vi "Non_empty_judgment.vi"(0 "TEMP":string, 1 "HN":string[](array[string]), 2 "生产日期":string, 3 "校准日期":string, 4 "核验员":string, 5 "HS":sgl[](array[numeric]), 6 "MODE":string, 7 "TV":sgl[][](array[numeric]), 8 "DIN":string, 9 "TESTS":sgl[][](array[numeric]), 10 "TSN":string, 11 "NAME":string) -> (16 "结果":bool)   [LabVIEW 2019]
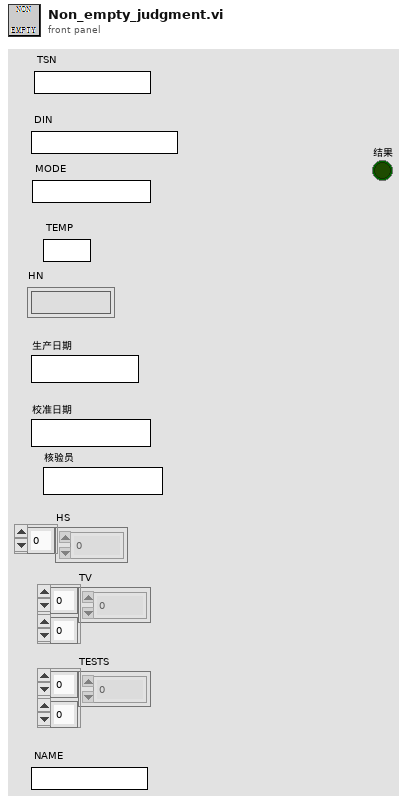
[diagram p1: front panel]
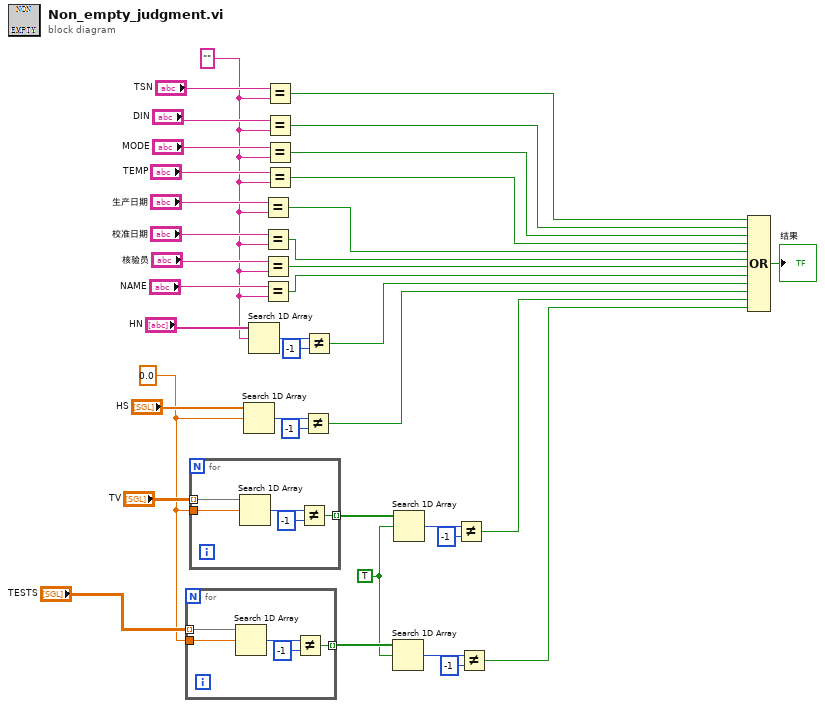
[diagram p0: block diagram]
diagram:
  w18 = TRUE
  w21 = 0.0
  w29 = ""
  n1 = for {
    tunnel: "TESTS" -> [w41] mode=indexing
    tunnel: w21 -> [w40]
    tunnel: [w39] -> w19 mode=indexing
    n2 = Search 1D Array(1D array=w41, element=w40) -> (index of element=w42:i32)  [unwired: 1 in]
    n3 = Not Equal?(x=w42, y=-1) -> (x != y?=w39:bool)
  }
  n4 = for {
    tunnel: "TV" -> [w46] mode=indexing
    tunnel: w21 -> [w45]
    tunnel: [w44] -> w20 mode=indexing
    n5 = Search 1D Array(1D array=w46, element=w45) -> (index of element=w47:i32)  [unwired: 1 in]
    n6 = Not Equal?(x=w47, y=-1) -> (x != y?=w44:bool)
  }
  n7 = Search 1D Array(1D array="HS", element=w21) -> (index of element=w24:i32)  [unwired: 1 in]
  n8 = Search 1D Array(1D array="HN", element=w29) -> (index of element=w28:i32)  [unwired: 1 in]
  n9 = Equal?(x="生产日期", y=w29) -> (x = y?=w9:bool)
  n10 = Equal?(x="校准日期", y=w29) -> (x = y?=w8:bool)
  n11 = Equal?(x="核验员", y=w29) -> (x = y?=w7:bool)
  n12 = Equal?(x="NAME", y=w29) -> (x = y?=w6:bool)
  n13 = Equal?(x="TSN", y=w29) -> (x = y?=w13:bool)
  n14 = Equal?(x="DIN", y=w29) -> (x = y?=w12:bool)
  n15 = Equal?(x="MODE", y=w29) -> (x = y?=w11:bool)
  n16 = Equal?(x="TEMP", y=w29) -> (x = y?=w10:bool)
  n17 = Not Equal?(x=w24, y=-1) -> (x != y?=w4:bool)
  n18 = Not Equal?(x=w28, y=-1) -> (x != y?=w5:bool)
  n19 = Search 1D Array(1D array=w19, element=w18) -> (index of element=w14:i32)  [unwired: 1 in]
  n20 = Search 1D Array(1D array=w20, element=w18) -> (index of element=w17:i32)  [unwired: 1 in]
  n21 = Not Equal?(x=w17, y=-1) -> (x != y?=w3:bool)
  n22 = Not Equal?(x=w14, y=-1) -> (x != y?=w2:bool)
  n23 = Compound Arithmetic op=OR(w13, w12, w11, w10, w9, w8, w7, w6, w5, w4, w3, w2) -> (→"结果":bool)
